vi "get_input.vi"(0 "Offline queue":refnum<queue>, 5 "Read queue":refnum<queue>, 7 "Offline options":T1 {"Range" min=0 step=1}, 9 "Time Stamp in":timestamp, 12 "Always display":bool) -> (4 "timed out?":bool, 6 "Input data":waveform(dbl)[][](array[waveform]), 8 "Current":i32, 10 "Time Stamp out":timestamp, 14 "Display update":bool, 15 "Replaying":bool)   [LabVIEW 2014]
uses:
  offline_options.ctl
panel:
  # "If true, don't suppress display update when there is input backlog."
  # "Start"
  # "End"
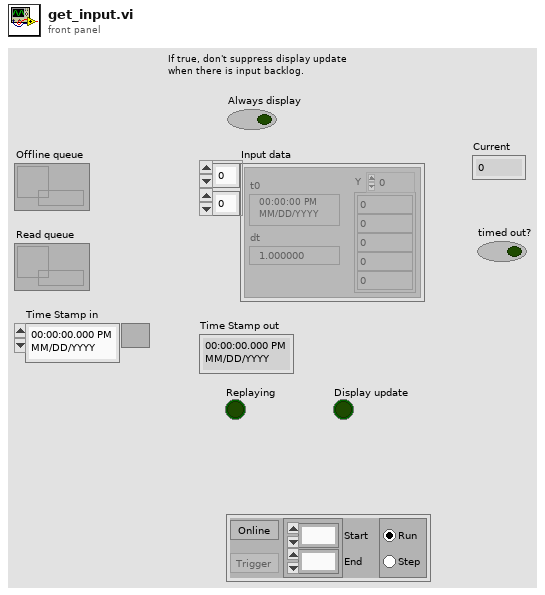
[diagram p1: front panel]
types:
  T1 = typedef "offline_options.ctl" = cluster{"Offline":bool, "Trigger":bool, "Range":i32[], "Run mode":enum32{"Run", "Step"}}
  T2 = cluster{"Range":i32[], "Run mode":enum32{"Run", "Step"}}
  T3 = cluster{"Vector of waveforms":waveform(dbl)[][]}[]
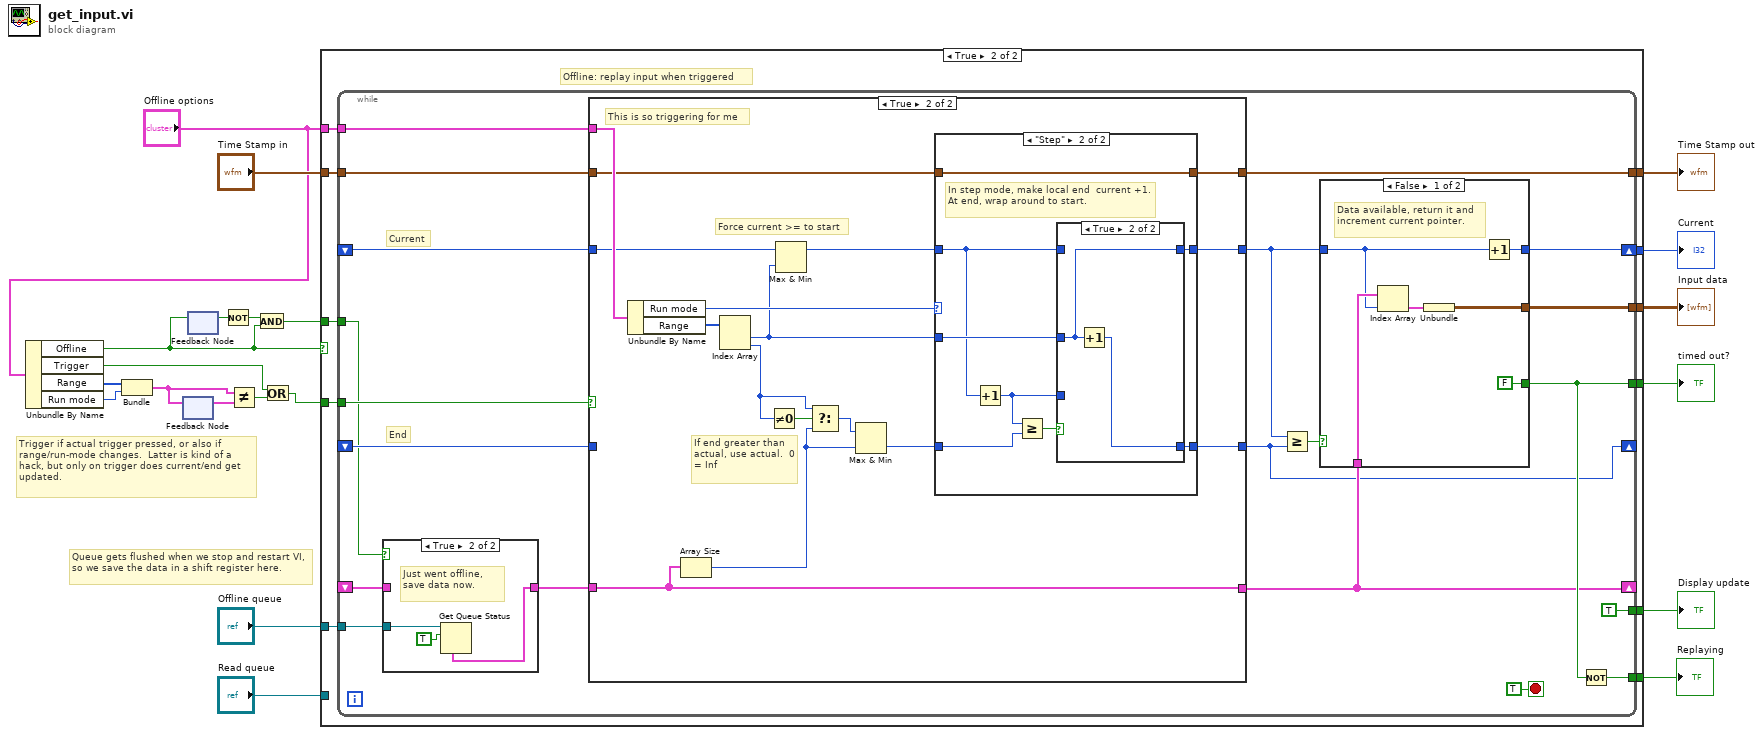
[diagram p0: block diagram]
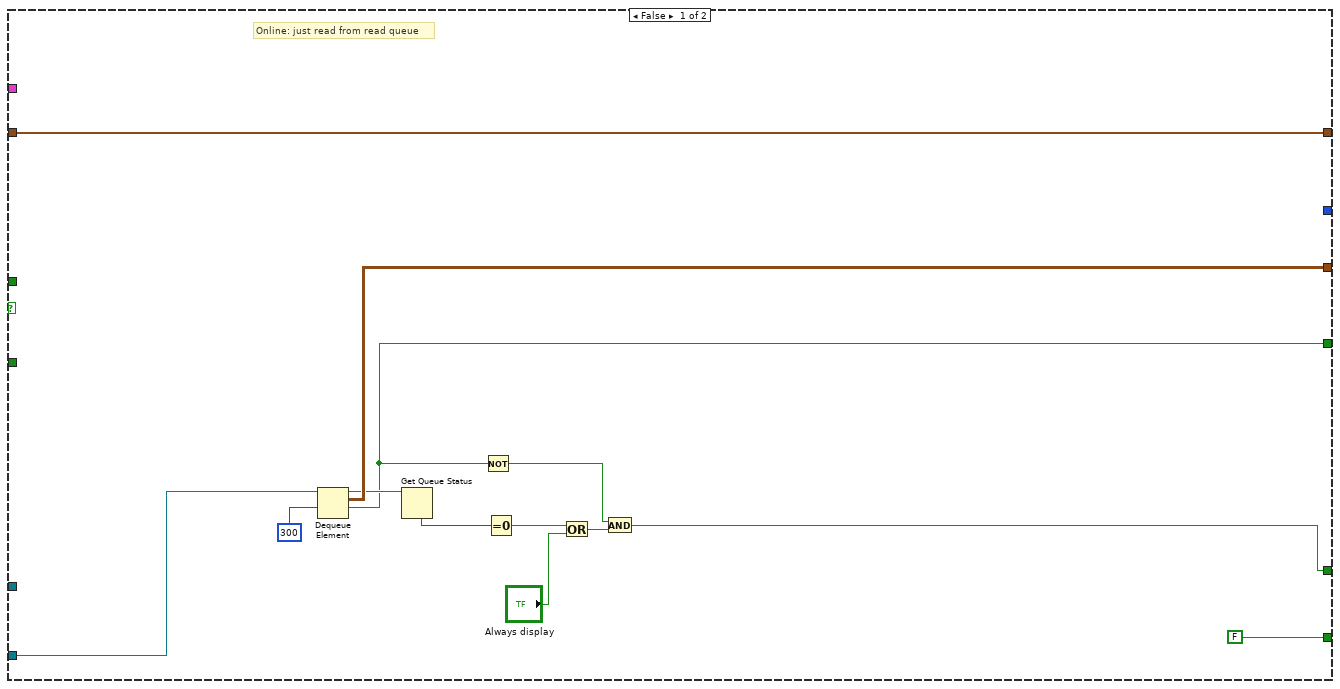
[diagram p2: hidden frame]
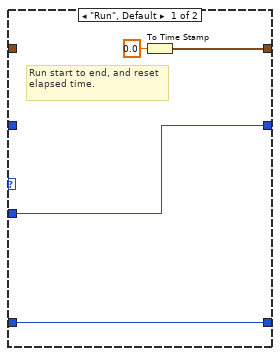
[diagram p5: hidden frame]
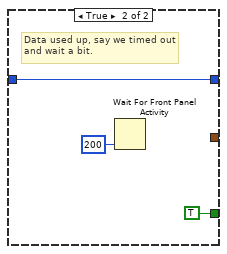
[diagram p7: hidden frame]
diagram:
  # "Queue gets flushed when we stop and restart VI, so we save the data in a shift register here."
  # "Trigger if actual trigger pressed, or also if range/run-mode changes.  Latter is kind of a hack, but only on trigger does current/end get updated."
  n1 = Unbundle By Name("Offline options") -> ("Offline"=w2:bool, "Trigger"=w11:bool, "Range"=w8:i32[], "Run mode"=w7:enum32{"Run", "Step"})
  n2 = Bundle("Range"=w8, "Run mode"=w7) -> (w6:T2)  [unwired: 1 in]
  n3 = feedback-in #1(w6) -> ()
  n4 = feedback #1() -> (w12:T2)  [unwired: 1 in]
  n5 = feedback #2() -> (w4:bool)  [unwired: 1 in]
  n6 = feedback-in #2(w2) -> ()
  n7 = Not(x=w4) -> (.not. x?=w3:bool)
  n8 = Not Equal?(x=w6, y=w12) -> (x != y?=w10:bool)
  n9 = And(x=w3, y=w2) -> (x .and. y?=w1:bool)
  n10 = Or(x=w11, y=w10) -> (x .or. y?=w9:bool)
  n11 = case shown="True" w2 {
    tunnel: "Read queue" -> [w34 _]
    tunnel: [w33 w40] -> w18
    tunnel: [w27 w41] -> w16
    tunnel: "Offline queue" -> [_ w45]
    tunnel: w9 -> [_ w44]
    tunnel: "Time Stamp in" -> [w31 w42]
    tunnel: [w31 w43] -> w21
    tunnel: [w26 w39] -> w15
    tunnel: [FALSE ("timed out?") w38] -> w14
    tunnel: "Offline options" -> [_ w37]
    tunnel: [_ w36] -> w13
    tunnel: w1 -> [_ w35]
    frame False {
      # "Online: just read from read queue"
      n12 = Dequeue Element(queue=w34, timeout in ms (-1)=300) -> (queue out=w29:refnum<queue>, element=w33:waveform(dbl)[][], timed out?=w27:bool)  [unwired: 1 in, 1 out]
      n13 = Get Queue Status(queue=w29) -> (# elements in queue=w25:i32)  [unwired: 2 in, 7 out]
      n14 = Not(x=w27) -> (.not. x?=w28:bool)
      n15 = Equal To 0?(x=w25) -> (x = 0?=w24:bool)
      n16 = Or(x=w24, y="Always display") -> (x .or. y?=w23:bool)
      n17 = And(x=w28, y=w23) -> (x .and. y?=w26:bool)
    }
    frame True {
      # "Offline: replay input when triggered"
      n18 = while {
        tunnel: w45 -> [w47]
        tunnel: w44 -> [w61]
        tunnel: [w59] -> w43
        shift-right: [w52] -> _
        shift-left: _ -> [w48]
        shift-right: [w64] -> w36
        shift-left: _ -> [w58]
        tunnel: w42 -> [w60]
        tunnel: [w55] -> w41
        tunnel: [w63] -> w40
        tunnel: [TRUE] -> w39
        tunnel: [w54] -> w38
        tunnel: w37 -> [w53]
        shift-right: [w50] -> _
        shift-left: _ -> [w51]
        tunnel: w35 -> [w49]
        stop <- TRUE stop-if-true
        # "End"
        # "Current"
        n19 = case shown="True" w49 {
          tunnel: w48 -> [w66 _]
          tunnel: w47 -> [_ w69]
          tunnel: [w66 w68] -> w46
          frame False {
          }
          frame True {
            # "Just went offline, save data now."
            n20 = Get Queue Status(queue=w69, return elements? (F)=TRUE) -> (elements=w68:T3)  [unwired: 1 in, 7 out]
          }
        }
        n21 = case shown="True" w61 {
          tunnel: w60 -> [w71 w82]
          tunnel: [w71 w89] -> w59
          tunnel: w58 -> [w73 w81]
          tunnel: [w73 w88] -> w57
          tunnel: [w72 w74] -> w52
          tunnel: w46 -> [w72 w74]
          tunnel: w53 -> [_ w87]
          tunnel: [w70 w76] -> w50
          tunnel: w51 -> [w70 _]
          frame False {
            # "Not triggered"
          }
          frame True {
            # "This is so triggering for me"
            # "Force current >= to start"
            # "If end greater than actual, use actual.  0 = Inf"
            n22 = Unbundle By Name(w87) -> ("Run mode"=w83:enum32{"Run", "Step"}, "Range"=w86:i32[])
            n23 = Array Size(array=w74) -> (size(s)=w84:i32)
            n24 = Index Array(array=w86) -> (element #1=w79:i32, element #2=w77:i32)  [unwired: 2 in]
            n25 = Not Equal To 0?(x=w77) -> (x != 0?=w85:bool)
            n26 = Max & Min(x=w81, y=w79) -> (max(x,y)=w80:i32)  [unwired: 1 out]
            n27 = Select(t=w77, s=w85, f=w84) -> (s? t:f=w78:i32)
            n28 = Max & Min(x=w78, y=w84) -> (min(x,y)=w75:i32)  [unwired: 1 out]
            n29 = case shown="\"Step\"" w83 {
              tunnel: [w92 w101] -> w89
              tunnel: [w91 w96] -> w88
              tunnel: w82 -> [_ w101]
              tunnel: w80 -> [_ w94]
              tunnel: w79 -> [w91 w98]
              tunnel: [w90 w97] -> w76
              tunnel: w75 -> [w90 w100]
              frame "Run", Default {
                # "Run start to end, and reset elapsed time."
                n30 = To Time Stamp(1:0.0 ("Fs low")) -> (0:w92:timestamp)
              }
              frame "Step" {
                # "In step mode, make local end  current +1.  At end, wrap around to start."
                n31 = Increment(x=w94) -> (x+1=w95:i32)
                n32 = Greater Or Equal?(x=w95, y=w100) -> (x >= y?=w99:bool)
                n33 = case shown="True" w99 {
                  tunnel: w98 -> [_ w104]
                  tunnel: [w103 w105] -> w97
                  tunnel: [w102 w104] -> w96
                  tunnel: w95 -> [w103 _]
                  tunnel: w94 -> [w102 _]
                  frame False {
                  }
                  frame True {
                    n34 = Increment(x=w104) -> (x+1=w105:i32)
                  }
                }
              }
            }
          }
        }
        n35 = Greater Or Equal?(x=w57, y=w50) -> (x >= y?=w62:bool)
        n36 = case shown="False" w62 {
          tunnel: [FALSE TRUE] -> w55
          tunnel: w57 -> [w107 w113]
          tunnel: [w111 w113] -> w64
          tunnel: w52 -> [w110 _]
          tunnel: [w108 _] -> w63
          frame False {
            # "Data available, return it and increment current pointer."
            n37 = Index Array(array=w110, index=w107) -> (element=w109:cluster{"Vector of waveforms":waveform(dbl)[][]})
            n38 = Unbundle(w109) -> ("Vector of waveforms"=w108:waveform(dbl)[][])
            n39 = Increment(x=w107) -> (x+1=w111:i32)
          }
          frame True {
            # "Data used up, say we timed out and wait a bit."
            n40 = Wait For Front Panel Activity(1:200 ("timeout ms (-1 never timeout)")) -> ()  [unwired: 2 in, 1 out]
          }
        }
        n41 = Not(x=w55) -> (.not. x?=w54:bool)
      }
    }
  }
  "Time Stamp out" <- w21
  "timed out?" <- w16
  "Input data" <- w18
  "Replaying" <- w14
  "Display update" <- w15
  "Current" <- w13
